vi "Reload Config.vi"(8 "error in (no error)":errorcluster, 9 "Promise":refnum<class "Promise.lvclass">, 10 "Config Type":string, 11 "Reconfigurable in":refnum<class "Reconfigurable.lvclass">) -> (0 "error out":errorcluster, 3 "Reconfigurable out":refnum<class "Reconfigurable.lvclass">)   [LabVIEW 2020, in "Volatus.lvlib" / "Reconfigurable.lvclass"]
uses:
  Reconfigurable.lvclass
  lv-promises/Promises/Promise/Promise.lvclass
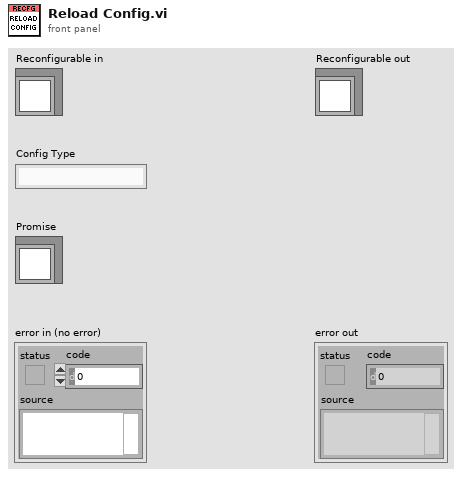
[diagram p1: front panel]
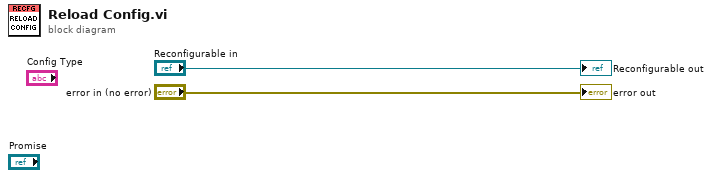
[diagram p0: block diagram]
diagram:
  "error out" <- "error in (no error)"
  "Reconfigurable out" <- "Reconfigurable in"
